vi "Create Class (Base).vi"() -> (4 "reference fpga":refnum<class "niUSRP Reference FPGA v1.lvclass">)   [LabVIEW 2025, in "niUSRP Reference FPGA v1.lvclass"]
uses:
  niUSRP Reference FPGA v1.lvclass
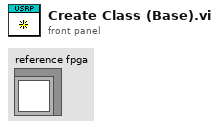
[diagram p1: front panel]
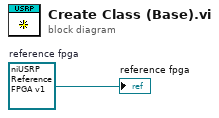
[diagram p0: block diagram]
diagram:
  w1 = refnum<class "niUSRP Reference FPGA v1.lvclass"> refnum  # reference fpga
  "reference fpga" <- w1
